vi "Get Motor Name.vi"(8 "error in (no error)":errorcluster, 11 "motor communication in":refnum<class "NI_Robotics_Motor Communication.lvclass">) -> (0 "error out":errorcluster, 2 "motor name":string, 3 "motor communication out":refnum<class "NI_Robotics_Motor Communication.lvclass">)   [LabVIEW 2017, in "NI_Robotics_Motor Communication.lvclass"]
uses:
  <vilib>/robotics/Actuation/Motor Communication/NI_Robotics_Motor Communication.lvclass
  <vilib>/robotics/Actuation/Motor Communication/NI_Robotics_Motor Communication.lvclass/NI_Robotics_Motor Communication.ctl
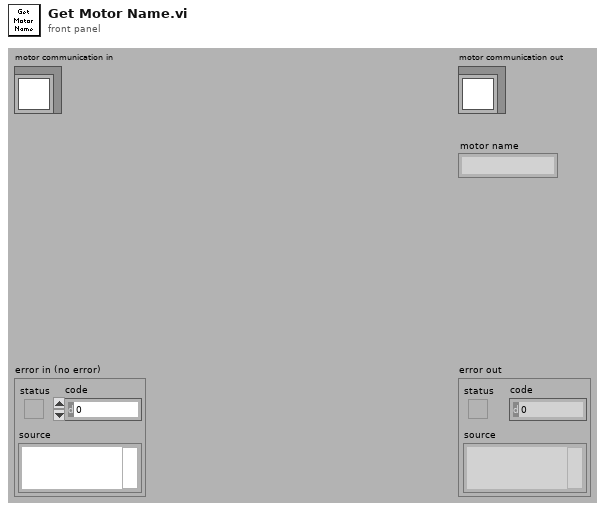
[diagram p1: front panel]
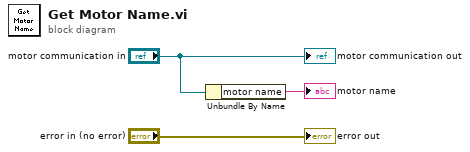
[diagram p0: block diagram]
diagram:
  n1 = Unbundle By Name("motor communication in") -> ("motor name"=→"motor name":string)
  "error out" <- "error in (no error)"
  "motor communication out" <- "motor communication in"
